vi "Blink.vi"() -> ()   [LabVIEW 2010]
doc: "This example shows how to control one of the Red Pitaya on board LEDs and make it blink."
uses:
  RedPitaya.lvlib
panel:
  in  "LED #":string(combo)="LED5"
  in  "ms to wait":u32=1000
  in  "IP address":string="192.168.4.129"
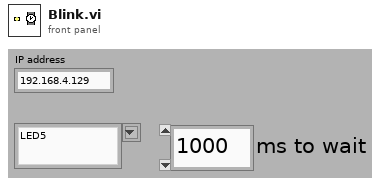
[diagram p1: front panel]
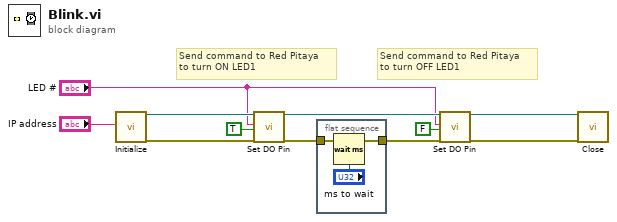
[diagram p0: block diagram]
diagram:
  # "Send command to Red Pitaya\nto turn OFF LED1"
  # "Send command to Red Pitaya\nto turn ON LED1"
  n1 = call "Initialize.vi"("IP address"="IP address") -> ("RedPitaya TCP Connection"=w11:refnum<k5>, "error out"=w10:errorcluster)  [unwired: 17 in]
  n2 = call "Set DO Pin.vi"("RedPitaya connection in"=w11, "Pin #"="LED #", "State"=TRUE, "error in"=w10) -> ("RedPitaya connection out"=w7:refnum<k5>, "error out"=w6:errorcluster)  [unwired: 14 in]
  n3 = flat-sequence {
    tunnel: w6 -> [w13]
    tunnel: [w13] -> w5
    frame #0 {
      n4 = Wait (ms)(milliseconds to wait="ms to wait") -> ()  [unwired: 1 out]
    }
  }
  n5 = call "Set DO Pin.vi"("RedPitaya connection in"=w7, "Pin #"="LED #", "State"=FALSE, "error in"=w5) -> ("RedPitaya connection out"=w9:refnum<k5>, "error out"=w8:errorcluster)  [unwired: 14 in]
  n6 = call "Close.vi"("connection ID"=w9, "error in"=w8) -> ()  [unwired: 17 in, 1 out]
